vi "Consumer.vi"(8 "error in (no error)":errorcluster, 9 "Data":variant, 10 "Case ID":string, 11 "Tamer in":refnum<class "Tamer.lvclass">=refnum) -> (0 "error out":errorcluster, 3 "Tamer out":refnum<class "Tamer.lvclass">)   [LabVIEW 2020, in "CIRCUS_uServices.lvlib" / "Tamer.lvlib" / "Tamer.lvclass"]
uses:
  Tamer.lvclass
  Tamer Consumer Case Selector.ctl
  Run Utilities/TypeDefs/Messages/Schedule Message - Standard.ctl
  Run Utilities/Run Utilities.lvlib
  Run Utilities/TypeDefs/Return Code.ctl
  Run Utilities/TypeDefs/Messages/Banana Message.ctl
  Internatl Banana.ctl
  Tamer GV.vi
  TALOS/TALOS_PPL.lvlibp
  TALOS/TALOS_PPL.lvlibp/Father of all uServices/Father of all uServices/Father of all uServices.lvclass
  TALOS/TALOS_PPL.lvlibp/Guardian/Guardian/Requests.ctl
  TALOS/TALOS_PPL.lvlibp/Guardian/Guardian/Guardian.lvclass
  TALOS/TALOS_PPL.lvlibp/Ancestor/Ancestor/Infinite Message Selector.ctl
  TALOS/TALOS_PPL.lvlibp/Ancestor/Ancestor/Ancestor.lvclass
  TALOS/TALOS_PPL.lvlibp/Support VIs/Go-NoGo.ctl
  TALOS/TALOS_PPL.lvlibp/Support VIs/Global Constants.vi
  Run Utilities/TypeDefs/Messages/Monkey Status Message.ctl
  Run Utilities/TypeDefs/Monkey Status.ctl
  Run Utilities/TypeDefs/Script Checker Result.ctl
  Run Utilities/TypeDefs/Messages/Script Checker Message.ctl
  Run Utilities/TypeDefs/Synchronize FPGA Cluster.ctl
  Run Utilities/TypeDefs/Messages/Schedule Message - Parallel.ctl
  Stop Message.ctl
  Link Chain GUI.ctl
  Monkey Summary.ctl
  TALOS/TALOS_PPL.lvlibp/Father of all uServices/Father of all uServices/Children Methods/Get GUI Item Value - Variant.vi
  Run Utilities/Schedule/Schedule.lvclass
  C:/Users/marco/Documents/GitHub_Lab/CIRCUS/TALOS/TALOS_PPL.lvlibp/Father of all uServices/Father of all uServices/Father of all uServices.lvclass
  C:/Users/marco/Documents/GitHub_Lab/CIRCUS/TALOS/TALOS_PPL.lvlibp/Ancestor/Ancestor/Ancestor.lvclass
  C:/Users/marco/Documents/GitHub_Lab/CIRCUS/TALOS/Actor Framework.lvlibp/1abvi3w/vi.lib/ActorFramework/Actor/Actor.lvclass
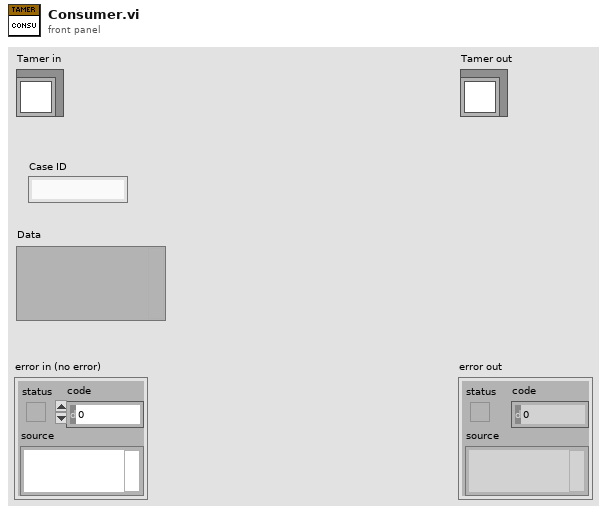
[diagram p1: front panel]
types:
  T1 = typedef "CIRCUS_uServices.lvlib/Tamer.lvlib/Tamer.lvclass/Tamer Consumer Case Selector.ctl" = enum16{"New schedule", "Initiate RUN", "Parse Schedules", "Script Checker", "Banana after Quality Check", "Update Crit Lvl", "Propagate Banana", "Reply from Guardian", "Reply from uService", "Timeout of RUN", "uService Replies Check", "Update from Monkey", "Monkey Died", "Reschedule", "Rerun", "Stop DAQ", "Stop Schedule", "Skip Run", "Kill Process", "Update GV"}
  T2 = typedef "CIRCUS_uServices.lvlib/Run Utilities.lvlib/Schedule Message - Standard.ctl" = cluster{"Schedules":refnum<class "Schedule.lvclass">[]}
  T3 = typedef "CIRCUS_uServices.lvlib/Run Utilities.lvlib/Schedule Message - Parallel.ctl" = cluster{"Schedules":refnum<class "Schedule.lvclass">[], "Synchronised":T4[]}
  T4 = typedef "CIRCUS_uServices.lvlib/Run Utilities.lvlib/Synchronize FPGA Cluster.ctl" = cluster{"Status":bool, "FPGA Name":string}
  T5 = typedef "TALOS_PPL.lvlibp/Guardian.lvlib/Guardian.lvclass/Requests.ctl" = enum16{"Ready to Launch", "Start RUN", "Stop RUN", "Update DAQ Params", "Update Error Listbox", "Update Run Status", "Update Kasli Log", "Run Stopped with Errors", "Switch uS View"}
  T6 = typedef "TALOS_PPL.lvlibp/Go-NoGo.ctl" = cluster{"ID":string, "Status":bool, "Data":string[], "GUID":string}
  T7 = typedef "CIRCUS_uServices.lvlib/Run Utilities.lvlib/Script Checker Message.ctl" = cluster{"Monkey ID":string, "Script Checker Result":T8}
  T8 = typedef "CIRCUS_uServices.lvlib/Run Utilities.lvlib/Script Checker Result.ctl" = enum16{"Passed", "Failed", "Empty"}
  T9 = typedef "CIRCUS_uServices.lvlib/Run Utilities.lvlib/Banana Message.ctl" = cluster{"FPGA Name":string, "Return Code":T10}
  T10 = typedef "CIRCUS_uServices.lvlib/Run Utilities.lvlib/Return Code.ctl" = enum16{"All Good", "Retry", "Skip", "Skip All", "ABORT"}
  T11 = typedef "CIRCUS_uServices.lvlib/Tamer.lvlib/Tamer.lvclass/Internatl Banana.ctl" = cluster{"Process ID":string, "Return Code":T10}
  T12 = typedef "CIRCUS_uServices.lvlib/Tamer.lvlib/Tamer.lvclass/Stop Message.ctl" = cluster{"Gracefully":bool, "Process":string}
  T13 = typedef "TALOS_PPL.lvlibp/Ancestor.lvlib/Ancestor.lvclass/Infinite Message Selector.ctl" = enum16{"Start", "Stop", "Check", "Flush (Stop all)", "Init"}
  T14 = typedef "CIRCUS_uServices.lvlib/Run Utilities.lvlib/Monkey Status Message.ctl" = cluster{"Monkey ID":string, "Monkey Status":T15, "Scripts left":u32, "ETA":string, "Current Action":string, "Report from previous RUNs":string, "Skipped RUNs":refnum<class "Schedule.lvclass">}
  T15 = typedef "CIRCUS_uServices.lvlib/Run Utilities.lvlib/Monkey Status.ctl" = enum16{"Init", "Paused", "Ongoing", "Stopped", "Finished (no errors)", "Finished (with errors)"}
  T16 = typedef "CIRCUS_uServices.lvlib/Tamer.lvlib/Tamer.lvclass/Monkey Summary.ctl" = cluster{"Color":u32, "Status":T15, "Continuous":bool, "Scripts left":u32, "Scripts skipped":u32, "ETA":string, "Current Action":string, "Report from previous RUNs":string, "Monkey ID":string, "With DAQ?":bool, "Linked?":T17, "Paused":bool}
  T17 = typedef "CIRCUS_uServices.lvlib/Tamer.lvlib/Tamer.lvclass/Link Chain GUI.ctl" = bool
  T18 = typedef "CIRCUS_uServices.lvlib/Tamer.lvlib/Tamer.lvclass/Tamer Status.ctl" = cluster{"Monkeys on the Stage":T16[], "All Monkeys Idle":bool}
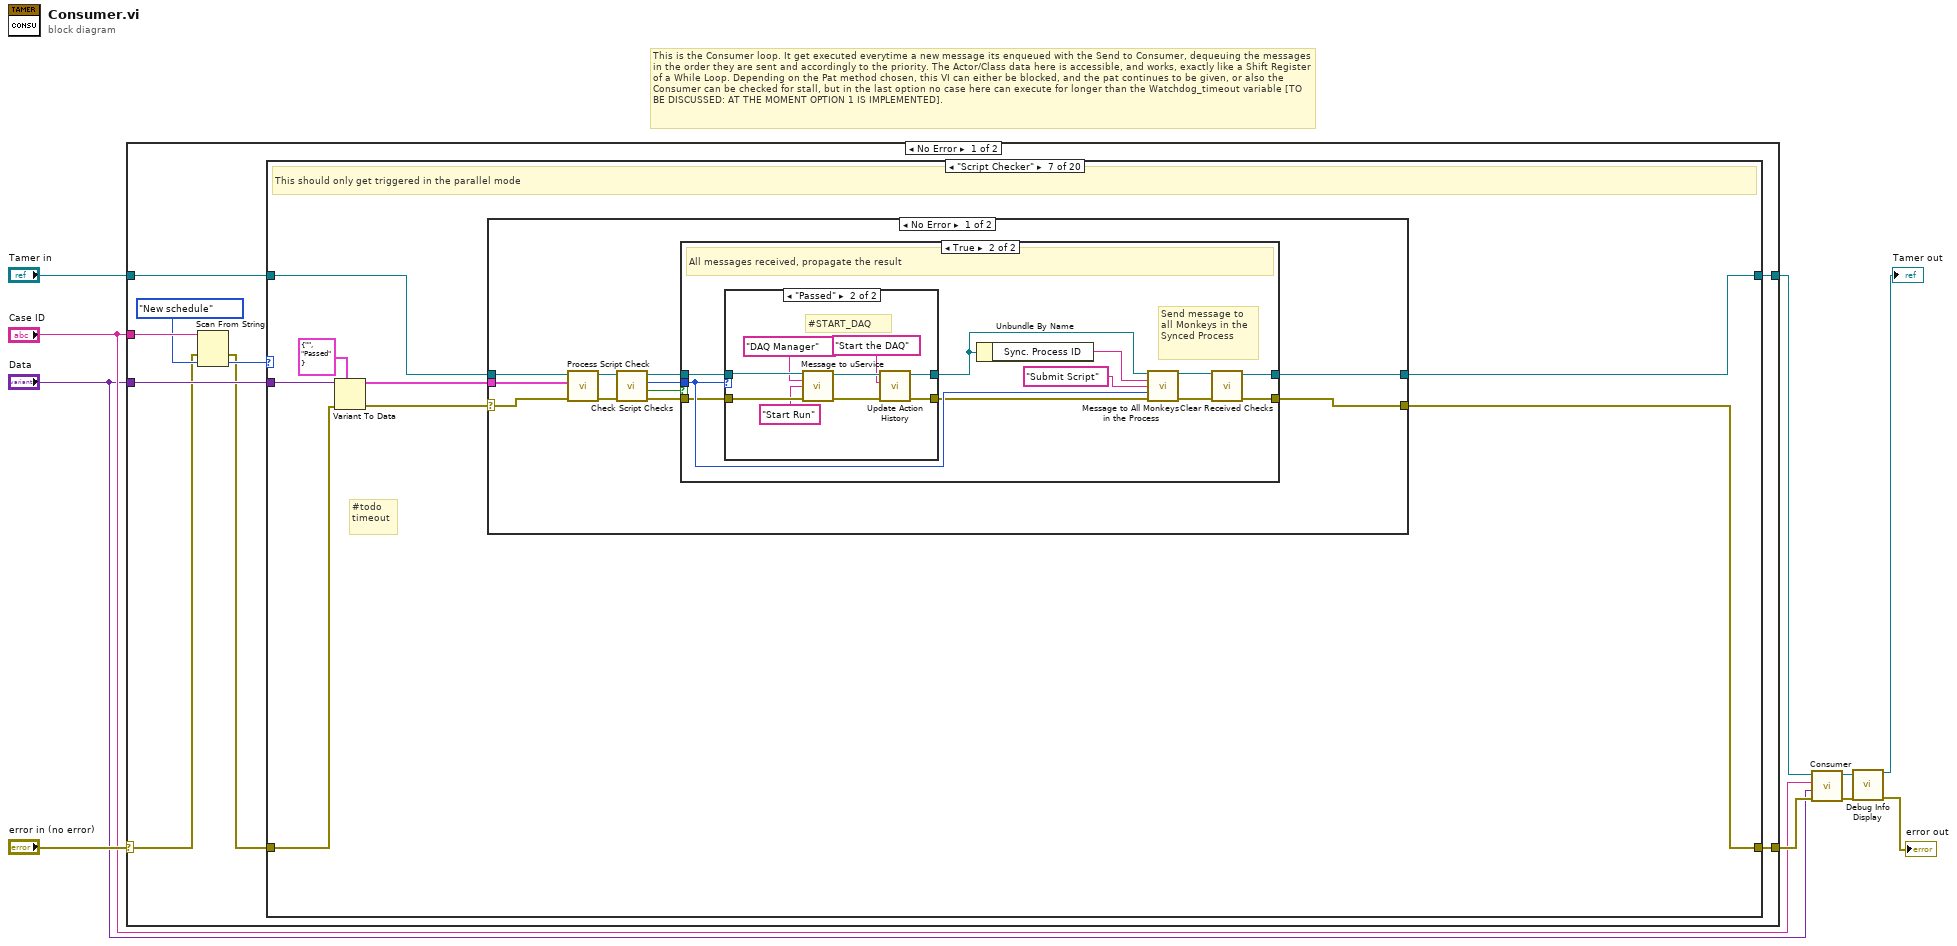
[diagram p0: block diagram]
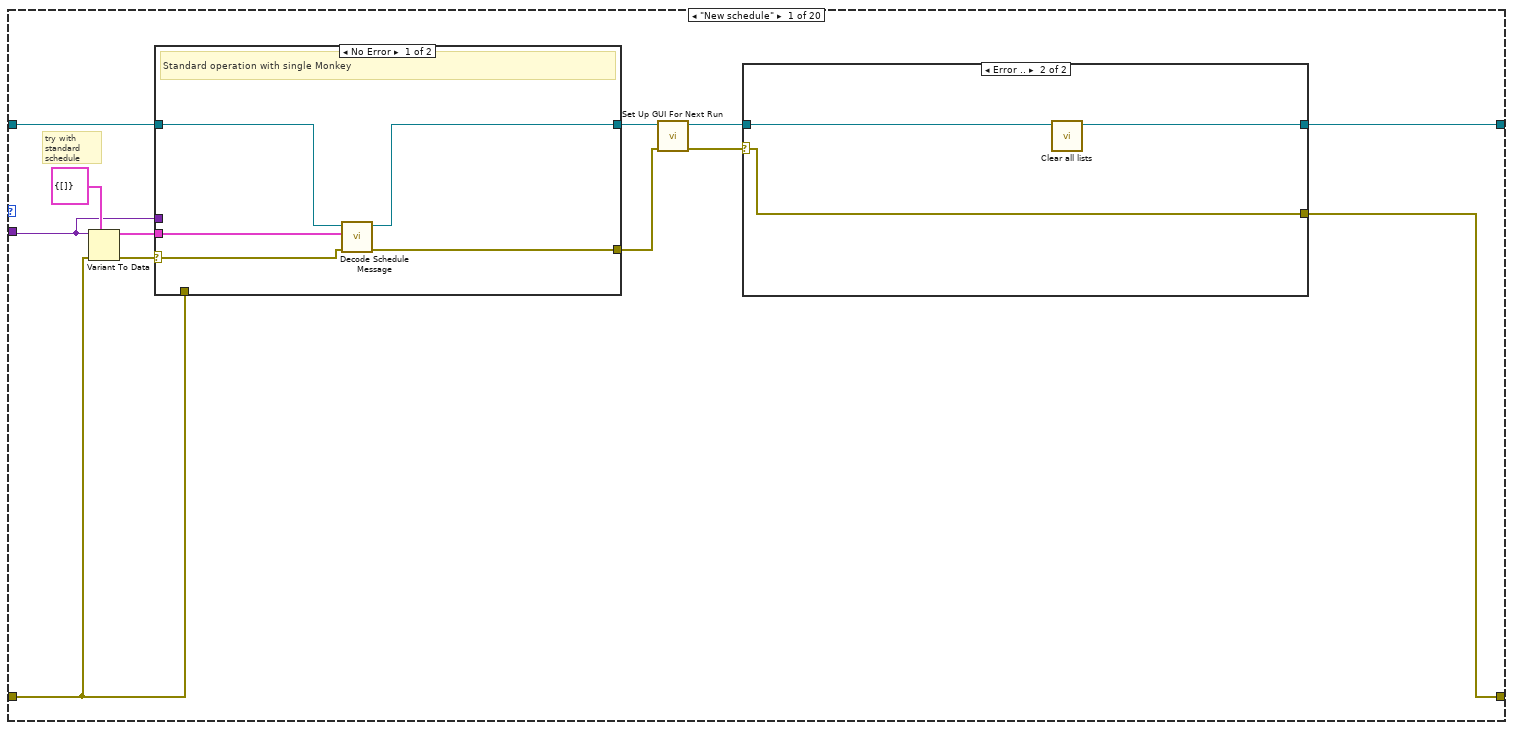
[diagram p2: hidden frame]
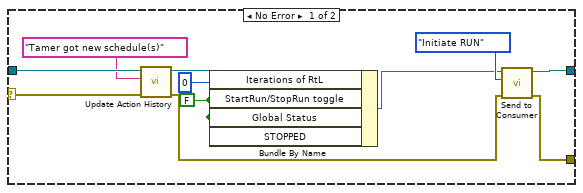
[diagram p3: hidden frame]
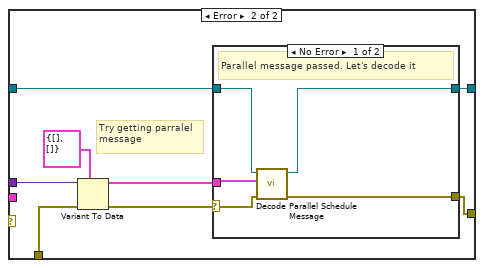
[diagram p4: hidden frame]
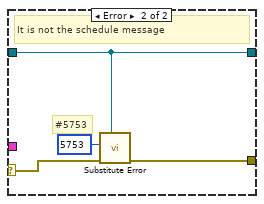
[diagram p5: hidden frame]
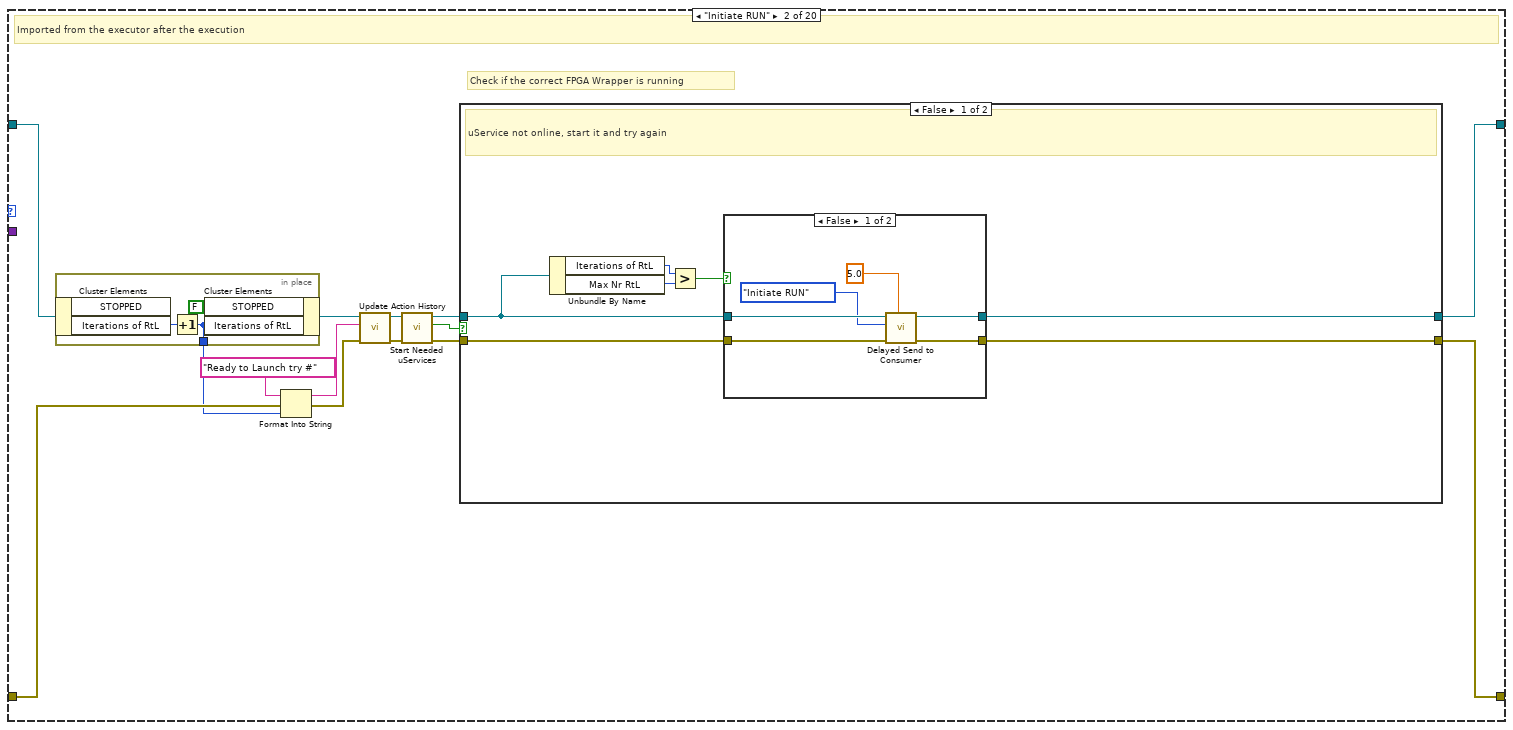
[diagram p6: hidden frame]
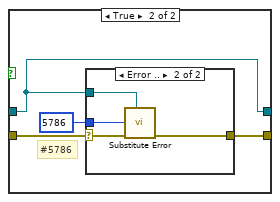
[diagram p7: hidden frame]
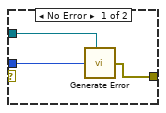
[diagram p8: hidden frame]
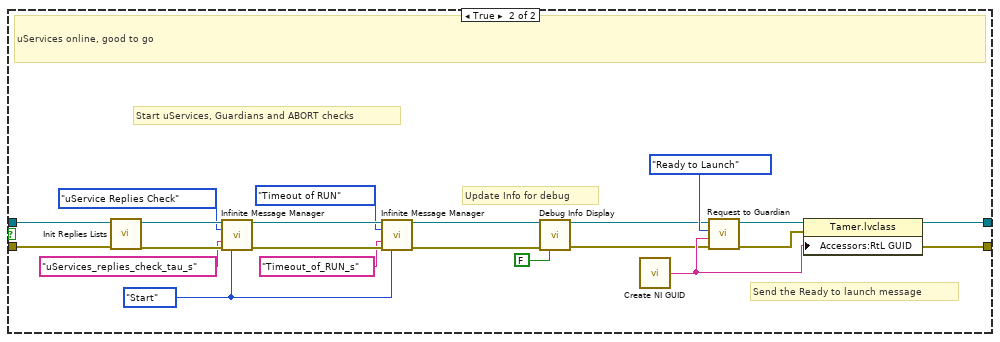
[diagram p9: hidden frame]
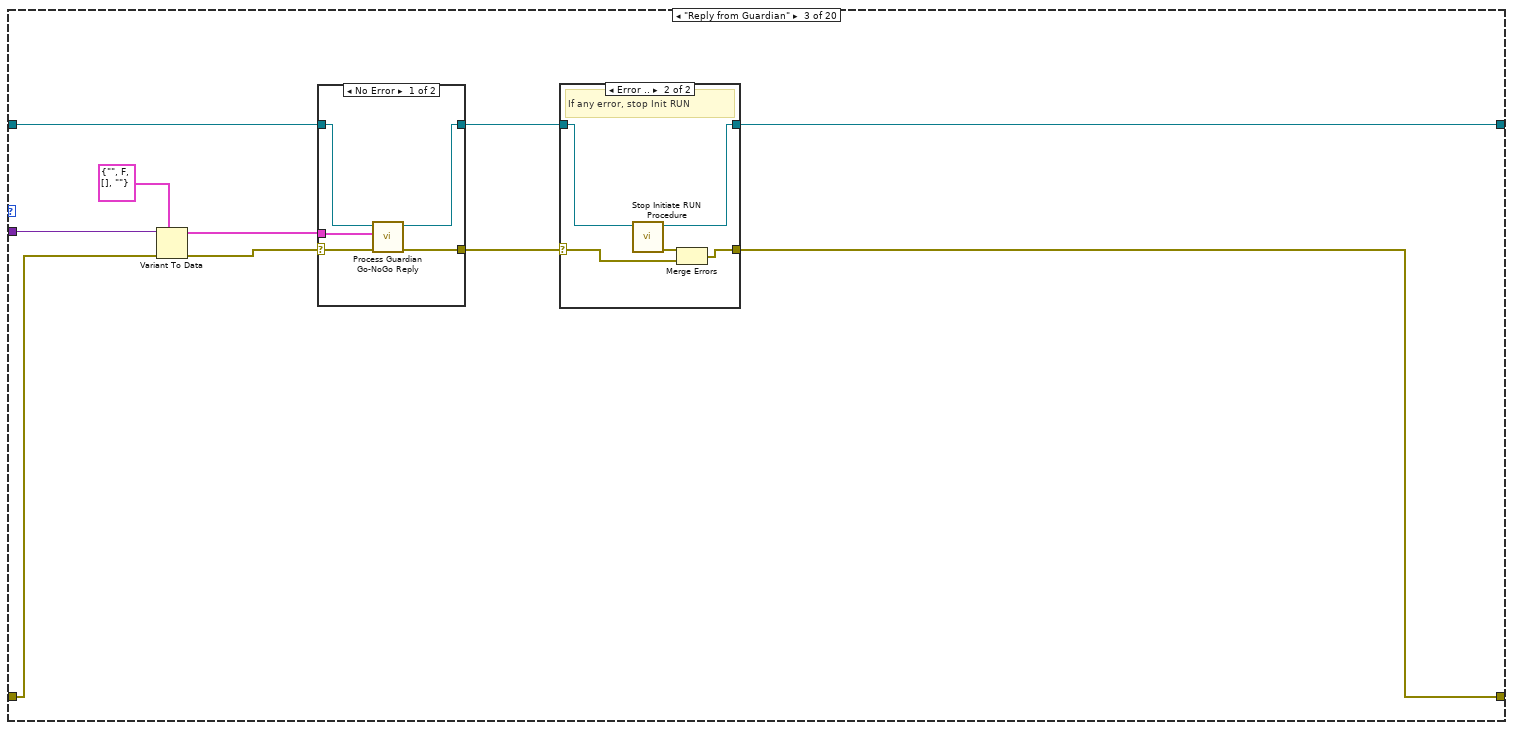
[diagram p10: hidden frame]
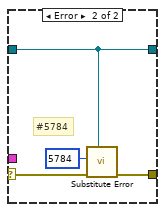
[diagram p12: hidden frame]
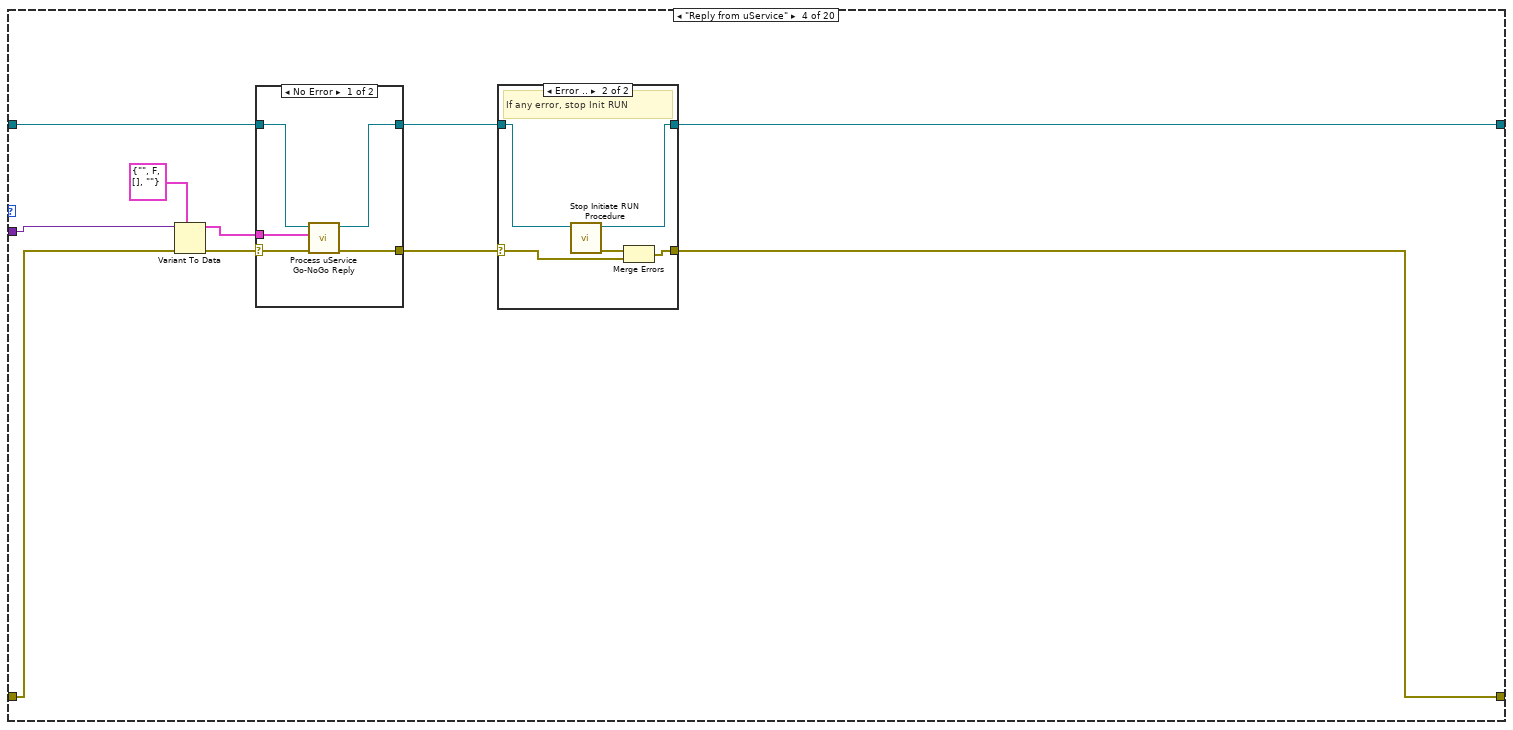
[diagram p13: hidden frame]
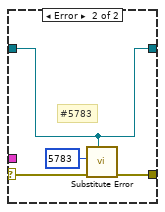
[diagram p15: hidden frame]
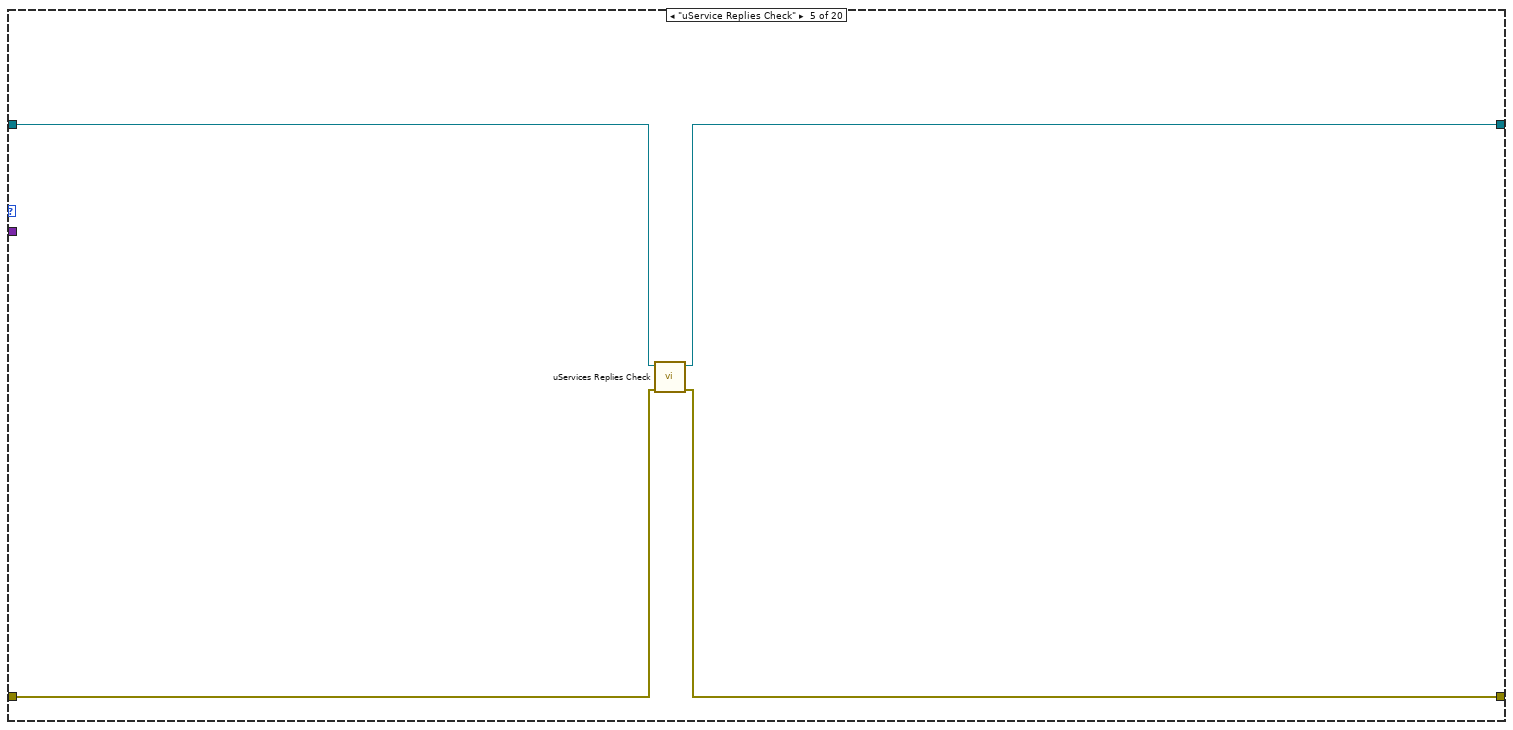
[diagram p16: hidden frame]
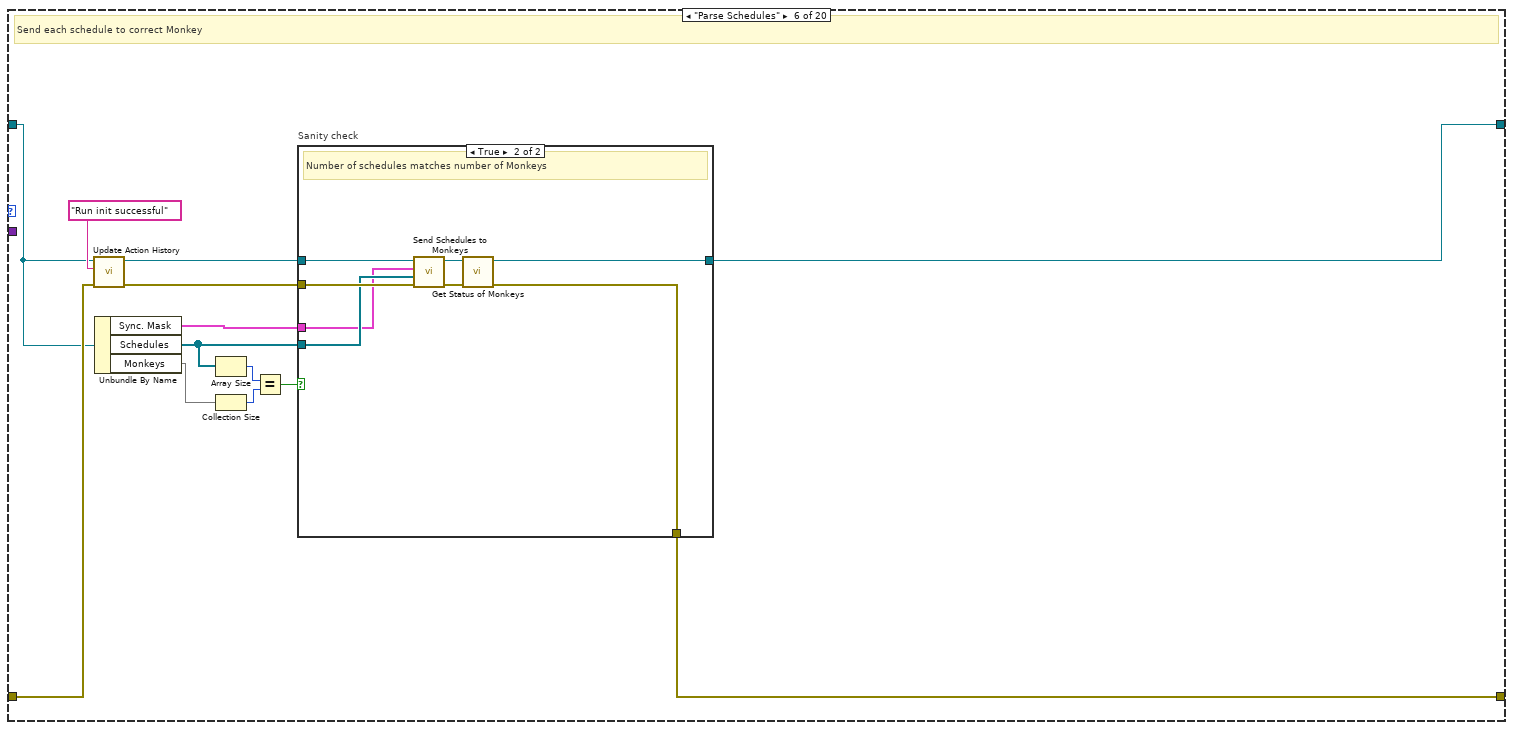
[diagram p17: hidden frame]
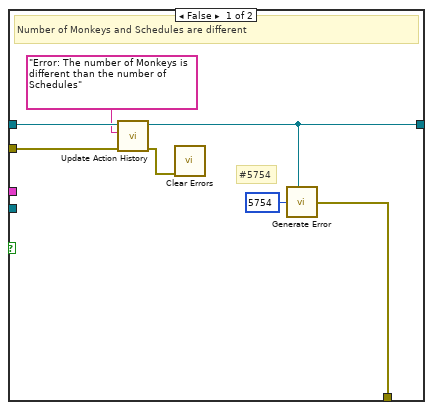
[diagram p18: hidden frame]
diagram:
  # "This is the Consumer loop. It get executed everytime a new message its enqueued with the Send to Consumer, dequeuing the messages in the order they are sent and accordingly to the priority. The Actor/Class data here is accessible, and works, exactly like a Shift Register of a While Loop. Depending on the Pat method chosen, this VI can either be blocked, and the pat continues to be given, or also the Consumer can be checked for stall, but in the last option no case here can execute for longer than the Watchdog_timeout variable [TO BE DISCUSSED: AT THE MOMENT OPTION 1 IS IMPLEMENTED]."
  n1 = case shown="No Error" "error in (no error)" {
    selector: "error in (no error)" -> [w12 w775]
    tunnel: [w18 w776] -> w7
    tunnel: "Tamer in" -> [w19 w776]
    tunnel: [w16 w775] -> w8
    tunnel: "Case ID" -> [w15 _]
    tunnel: "Data" -> [w17 _]
    frame No Error {
      n2 = Scan From String(input string=w15, error in=w12, default 1=Tamer_Consumer_Case_Selector."New schedule" ("Consumer Case Selector")) -> (error out=w11:errorcluster, output 1=w13:T1)  [unwired: 2 in, 2 out]
      n3 = case shown="\"Script Checker\"" w13 {
        tunnel: w19 -> [w26 w68 w136 w162 w183 w190 w217 w262 w329 w335 w354 w419 w435 w503 w543 w578 w627 w703 w767 w773]
        tunnel: [w21 w77 w135 w158 w184 w191 w215 w269 w328 w337 w364 w416 w437 w502 w562 w584 w631 w705 w764 w770] -> w18
        tunnel: w17 -> [w28 _ w134 w161 _ _ w222 w263 _ w341 w366 _ w440 w508 w549 w582 w632 w706 w763 _]
        tunnel: [w20 w76 w132 w159 w185 w197 w216 w268 w326 w336 w363 w417 w436 w501 w561 w586 w630 w704 w765 w769] -> w16
        tunnel: w11 -> [w27 w81 w133 w160 w186 w194 w220 w271 w327 w332 w365 w418 w438 w506 w550 w581 _ w707 w766 w772]
        frame "New schedule" {
          # "try with standard schedule"
          n4 = Variant To Data(error in=w27, type=T2 {"Schedules"=[]} ("Schedule message - parallel"), Variant=w28) -> (data=w29:T2, error out=w30:errorcluster)
          n5 = case shown="No Error" w30 {
            selector: w30 -> [w48 _]
            tunnel: w29 -> [w49 _]
            tunnel: w28 -> [_ w58]
            tunnel: w27 -> [_ w57]
            tunnel: w26 -> [w50 w53]
            tunnel: [w47 w52] -> w25
            tunnel: [w46 w51] -> w23
            frame No Error {
              # "Standard operation with single Monkey"
              n6 = call-dynamic "Decode Schedule Message.vi"("error in (no error)"=w48, "Schedule message"=w49, "Tamer in"=w50) -> ("error out"=w46:errorcluster, "Tamer out"=w47:refnum<class "Tamer.lvclass">)  [unwired: 7 in]
            }
            frame Error {
              # "Try getting parralel message"
              n7 = Variant To Data(error in=w57, type=T3 {"Schedules"=[], "Synchronised"=[]} ("Schedule message - parallel"), Variant=w58) -> (data=w54:T3, error out=w55:errorcluster)
              n8 = case shown="No Error" w55 {
                selector: w55 -> [w61 w66]
                tunnel: w54 -> [w63 _]
                tunnel: w53 -> [w62 w65]
                tunnel: [w60 w65] -> w52
                tunnel: [w59 w67] -> w51
                frame No Error {
                  # "Parallel message passed. Let's decode it"
                  n9 = call-dynamic "Decode Parallel Schedule Message.vi"("error in (no error)"=w61, "Schedule message - parallel"=w63, "Tamer in"=w62) -> ("error out"=w59:errorcluster, "Tamer out"=w60:refnum<class "Tamer.lvclass">)  [unwired: 7 in]
                }
                frame Error {
                  # "#5753"
                  # "It is not the schedule message"
                  n10 = call "Substitute Error.vi"("LabVIEW Object"=w65, "error in (no error)"=w66, "Error Code"=5753) -> ("error out"=w67:errorcluster)  [unwired: 8 in]
                }
              }
            }
          }
          n11 = call-dynamic "Set Up GUI For Next Run.vi"("error in (no error)"=w23, "Tamer in"=w25) -> ("error out"=w22:errorcluster, "Tamer out"=w24:refnum<class "Tamer.lvclass">)  [unwired: 8 in]
          n12 = case shown="Error .." w22 {
            selector: w22 -> [w37 w45]
            tunnel: [w34 w43] -> w21
            tunnel: w24 -> [w42 w44]
            tunnel: [w32 w45] -> w20
            frame No Error {
              w38 = FALSE ("StartRun/StopRun toggle")
              n13 = call-dynamic "Update Action History.vi"("error in (no error)"=w37, "Action"="Tamer got new schedule(s)", "Tamer in"=w42) -> ("error out"=w33:errorcluster, "Tamer out"=w40:refnum<class "Tamer.lvclass">)  [unwired: 7 in]
              n14 = Bundle By Name(cluster=w40, "Iterations of RtL"=u8 0, "StartRun/StopRun toggle"=w38, "Global Status"=w38, "STOPPED"=w38) -> (w35:refnum<class "Tamer.lvclass">)
              n15 = call "Send to Consumer.vi"("error in (no error)"=w33, "Case ID"=Tamer_Consumer_Case_Selector."Initiate RUN" ("Monkey Consumer Case Selector"), "uService Template in"=w35) -> ("error out"=w32:errorcluster, "uService Template out"=w34:refnum<class "Tamer.lvclass">)  [unwired: 7 in]
            }
            frame Error {
              n16 = call-dynamic "Clear all lists.vi"("Tamer in"=w44) -> ("Tamer out"=w43:refnum<class "Tamer.lvclass">)  [unwired: 9 in, 1 out]
            }
          }
        }
        frame "Initiate RUN" {
          # "Check if the correct FPGA Wrapper is running"
          # "Imported from the executor after the execution"
          n17 = in-place {
            in-place-border: [w82] -> w69
            n18 = in-place-cluster #1(w68) -> ("Iterations of RtL"=w84:u8)  [unwired: 1 out]
            n19 = Increment(x=w84) -> (x+1=w82:u8)
            n20 = in-place-cluster #1("STOPPED"=FALSE, "Iterations of RtL"=w82) -> (w73:refnum<class "Tamer.lvclass">)
          }
          n21 = Format Into String(initial string="Ready to Launch try #", error in=w81, w69) -> (resulting string=w71:string, error out=w70:errorcluster)  [unwired: 1 in]
          n22 = call-dynamic "Update Action History.vi"("error in (no error)"=w70, "Action"=w71, "Tamer in"=w73) -> ("error out"=w74:errorcluster, "Tamer out"=w75:refnum<class "Tamer.lvclass">)  [unwired: 7 in]
          n23 = call-dynamic "Start Needed uServices.vi"("error in (no error)"=w74, "Tamer in"=w75) -> ("error out"=w79:errorcluster, "All online?"=w80:bool, "Tamer out"=w78:refnum<class "Tamer.lvclass">)  [unwired: 7 in]
          n24 = case shown="False" w80 {
            tunnel: w79 -> [w89 w112]
            tunnel: w78 -> [w88 w113]
            tunnel: [w91 w115] -> w77
            tunnel: [w90 w114] -> w76
            frame False {
              # "uService not online, start it and try again"
              n25 = Unbundle By Name(w88) -> ("Iterations of RtL"=w87:u8, "Max Nr RtL"=w86:u8)
              n26 = Greater?(x=w87, y=w86) -> (0:w85:bool)
              n27 = case shown="False" w85 {
                tunnel: [w97 w99] -> w91
                tunnel: [w96 w100] -> w90
                tunnel: w88 -> [w95 w99]
                tunnel: w89 -> [w94 w101]
                frame False {
                  n28 = call "Delayed Send to Consumer.vi"("Seconds (5)"=5.0 ("Delay"), "error in (no error)"=w94, "Case ID"=Tamer_Consumer_Case_Selector."Initiate RUN" ("Tamer Consumer Case Selector"), "Father of all uServices in"=w95) -> ("error out"=w96:errorcluster, "Father of all uServices out"=w97:refnum<class "Tamer.lvclass">)  [unwired: 6 in]
                }
                frame True {
                  # "#5786"
                  n29 = case shown="Error .." w101 {
                    selector: w101 -> [_ w108]
                    tunnel: [w102 w107] -> w100
                    tunnel: w99 -> [w104 w106]
                    tunnel: 5786 -> [w103 w105]
                    frame No Error {
                      n30 = call "Generate Error.vi"("Class"=w104, "Error Code"=w103) -> ("error out"=w102:errorcluster)  [unwired: 5 in]
                    }
                    frame Error {
                      n31 = call "Substitute Error.vi"("LabVIEW Object"=w106, "error in (no error)"=w108, "Error Code"=w105) -> ("error out"=w107:errorcluster)  [unwired: 8 in]
                    }
                  }
                }
              }
            }
            frame True {
              w123 = Infinite_Message_Selector."Start" ("Infinite Message Selector")
              # "Start uServices, Guardians and ABORT checks"
              # "Update Info for debug"
              # "Send the Ready to launch message"
              # "uServices online, good to go"
              n32 = call "Init Replies Lists.vi"("error in (no error)"=w112, "Monkey in"=w113) -> ("error out"=w127:errorcluster, "Monkey out"=w128:refnum<class "Tamer.lvclass">)  [unwired: 8 in]
              n33 = call-dynamic "Infinite Message Manager.vi"("Father of all uServices in"=w128, "Consumer Case Selector"=Tamer_Consumer_Case_Selector."uService Replies Check" ("Monkey Consumer Case Selector"), "Tau parameter"="uServices_replies_check_tau_s" ("SV Name"), "error in (no error)"=w127, "Infinite Message Selector"=w123) -> ("Father of all uServices out"=w125:refnum<class "Tamer.lvclass">, "error out"=w124:errorcluster)  [unwired: 8 in, 1 out]
              n34 = call-dynamic "Infinite Message Manager.vi"("Father of all uServices in"=w125, "Consumer Case Selector"=Tamer_Consumer_Case_Selector."Timeout of RUN" ("Monkey Consumer Case Selector"), "Tau parameter"="Timeout_of_RUN_s" ("SV Name"), "error in (no error)"=w124, "Infinite Message Selector"=w123) -> ("Father of all uServices out"=w119:refnum<class "Tamer.lvclass">, "error out"=w116:errorcluster)  [unwired: 8 in, 1 out]
              n35 = call-dynamic "Debug Info Display.vi"("Tamer in"=w119, "error in (no error)"=w116, "Do not clear"=FALSE) -> ("Tamer out"=w118:refnum<class "Tamer.lvclass">, "error out"=w117:errorcluster)  [unwired: 11 in]
              n36 = call <vilib>:"Create NI GUID.vi"() -> ("NI GUID"=w120:string)
              n37 = call "Request to Guardian.vi"("error in (no error)"=w117, "Data"=w120, "Requests"=Requests."Ready to Launch", "Father of all uServices in"=w118) -> ("error out"=w110:errorcluster, "Father of all uServices out"=w130:refnum<class "Tamer.lvclass">)  [unwired: 6 in]
              n38 = property class="Tamer.lvclass"(reference=w130, error in=w110, "Accessors:RtL GUID"=w120) -> (reference out=w115:refnum<class "Tamer.lvclass">, error out=w114:errorcluster)
            }
          }
        }
        frame "Reply from Guardian" {
          n39 = Variant To Data(error in=w133, type=T6 {"ID"="", "Status"=FALSE, "Data"=[], "GUID"=""} ("Go-NoGo"), Variant=w134) -> (data=w138:T6, error out=w139:errorcluster)
          n40 = case shown="No Error" w139 {
            selector: w139 -> [w152 w155]
            tunnel: [w151 w156] -> w140
            tunnel: w138 -> [w150 _]
            tunnel: w136 -> [w149 w153]
            tunnel: [w148 w153] -> w137
            frame No Error {
              n41 = call "Process Guardian Go-NoGo Reply.vi"("error in (no error)"=w152, "Go-NoGo"=w150, "Tamer in"=w149) -> ("error out"=w151:errorcluster, "Tamer out"=w148:refnum<class "Tamer.lvclass">)  [unwired: 7 in]
            }
            frame Error {
              # "#5784"
              n42 = call "Substitute Error.vi"("LabVIEW Object"=w153, "error in (no error)"=w155, "Error Code"=5784) -> ("error out"=w156:errorcluster)  [unwired: 8 in]
            }
          }
          n43 = case shown="Error .." w140 {
            selector: w140 -> [w142 w144]
            tunnel: [w142 w143] -> w132
            tunnel: [w141 w147] -> w135
            tunnel: w137 -> [w141 w146]
            frame No Error {
              # "All good!"
            }
            frame Error {
              # "If any error, stop Init RUN"
              n44 = call "Stop Initiate RUN Procedure.vi"("Tamer in"=w146) -> ("error out"=w145:errorcluster, "Tamer out"=w147:refnum<class "Tamer.lvclass">)  [unwired: 9 in]
              n45 = Merge Errors(w145, w144) -> (w143:errorcluster)
            }
          }
        }
        frame "Reply from uService" {
          n46 = Variant To Data(error in=w160, type=T6 {"ID"="", "Status"=FALSE, "Data"=[], "GUID"=""} ("Go-NoGo"), Variant=w161) -> (data=w166:T6, error out=w165:errorcluster)
          n47 = case shown="No Error" w165 {
            selector: w165 -> [w177 w181]
            tunnel: w166 -> [w178 _]
            tunnel: [w176 w182] -> w163
            tunnel: [w175 w179] -> w164
            tunnel: w162 -> [w174 w179]
            frame No Error {
              n48 = call "Process uService Go-NoGo Reply.vi"("error in (no error)"=w177, "Go-NoGo"=w178, "Tamer in"=w174) -> ("error out"=w176:errorcluster, "Tamer out"=w175:refnum<class "Tamer.lvclass">)  [unwired: 7 in]
            }
            frame Error {
              # "#5783"
              n49 = call "Substitute Error.vi"("LabVIEW Object"=w179, "error in (no error)"=w181, "Error Code"=5783) -> ("error out"=w182:errorcluster)  [unwired: 8 in]
            }
          }
          n50 = case shown="Error .." w163 {
            selector: w163 -> [w168 w169]
            tunnel: w164 -> [w167 w173]
            tunnel: [w168 w170] -> w159
            tunnel: [w167 w172] -> w158
            frame No Error {
              # "All good!"
            }
            frame Error {
              # "If any error, stop Init RUN"
              n51 = call "Stop Initiate RUN Procedure.vi"("Tamer in"=w173) -> ("error out"=w171:errorcluster, "Tamer out"=w172:refnum<class "Tamer.lvclass">)  [unwired: 9 in]
              n52 = Merge Errors(w171, w169) -> (w170:errorcluster)
            }
          }
        }
        frame "uService Replies Check" {
          n53 = call "uServices Replies Check.vi"("error in (no error)"=w186, "Tamer in"=w183) -> ("error out"=w185:errorcluster, "Tamer out"=w184:refnum<class "Tamer.lvclass">)  [unwired: 8 in]
        }
        frame "Parse Schedules" {
          # "Send each schedule to correct Monkey"
          n54 = call-dynamic "Update Action History.vi"("error in (no error)"=w194, "Action"="Run init successful", "Tamer in"=w190) -> ("error out"=w192:errorcluster, "Tamer out"=w195:refnum<class "Tamer.lvclass">)  [unwired: 7 in]
          n55 = Unbundle By Name(w190) -> ("Sync. Mask"=w199:T4[], "Schedules"=w198:refnum<class "Schedule.lvclass">[], "Monkeys"=w188:map{string, string[]})
          n56 = Array Size(array=w198) -> (size(s)=w189:i32)
          n57 = Collection Size(1:w188) -> (0:w187:i32)
          n58 = Equal?(x=w189, y=w187) -> (x = y?=w196:bool)
          n59 = case "Sanity check" shown="True" w196 {
            tunnel: w199 -> [_ w211]
            tunnel: w195 -> [w204 w213]
            tunnel: w198 -> [_ w212]
            tunnel: [w205 w207] -> w197
            tunnel: w192 -> [w203 w214]
            tunnel: [w200 w209] -> w191
            frame False {
              # "#5754"
              # "Number of Monkeys and Schedules are different"
              n60 = call-dynamic "Update Action History.vi"("error in (no error)"=w203, "Action"="Error: The number of Monkeys is different than the number of Schedules", "Tamer in"=w204) -> ("error out"=w201:errorcluster, "Tamer out"=w200:refnum<class "Tamer.lvclass">)  [unwired: 7 in]
              n61 = call <vilib>:"Clear Errors.vi"("error in (no error)"=w201) -> ()  [unwired: 5 in, 2 out]
              n62 = call "Generate Error.vi"("Class"=w200, "Error Code"=5754) -> ("error out"=w205:errorcluster)  [unwired: 5 in]
            }
            frame True {
              # "Number of schedules matches number of Monkeys"
              n63 = call "Send Schedules to Monkeys.vi"("error in (no error)"=w214, "Schedules"=w212, "Sync. Mask"=w211, "Tamer in"=w213) -> ("error out"=w208:errorcluster, "Tamer out"=w210:refnum<class "Tamer.lvclass">)  [unwired: 6 in]
              n64 = call-dynamic "Get Status of Monkeys.vi"("error in (no error)"=w208, "Tamer in"=w210) -> ("error out"=w207:errorcluster, "Tamer out"=w209:refnum<class "Tamer.lvclass">)  [unwired: 7 in, 1 out]
            }
          }
        }
        frame "Script Checker" {
          # "#todo\ntimeout"
          # "This should only get triggered in the parallel mode"
          n65 = Variant To Data(error in=w220, type=T7 {"Monkey ID"="", "Script Checker Result"=enum."Passed"} ("Message"), Variant=w222) -> (data=w218:T7, error out=w219:errorcluster)
          n66 = case shown="No Error" w219 {
            selector: w219 -> [w233 w261]
            tunnel: w218 -> [w224 _]
            tunnel: w217 -> [w225 w259]
            tunnel: [w223 w260] -> w216
            tunnel: [w226 w259] -> w215
            frame No Error {
              n67 = call-dynamic "Process Script Check.vi"("error in (no error)"=w233, "Message"=w224, "Tamer in"=w225) -> ("error out"=w231:errorcluster, "Tamer out"=w232:refnum<class "Tamer.lvclass">)  [unwired: 7 in]
              n68 = call-dynamic "Check Script Checks.vi"("error in (no error)"=w231, "Tamer in"=w232) -> ("error out"=w229:errorcluster, "Send Result?"=w230:bool, "Script Checker Result"=w228:T8, "Tamer out"=w227:refnum<class "Tamer.lvclass">)  [unwired: 6 in]
              n69 = case shown="True" w230 {
                tunnel: w229 -> [w234 w239]
                tunnel: w228 -> [_ w244]
                tunnel: w227 -> [w235 w238]
                tunnel: [w234 w241] -> w223
                tunnel: [w235 w240] -> w226
                frame False {
                  # "Waiting for some responses"
                }
                frame True {
                  # "Send message to all Monkeys in the Synced Process"
                  # "All messages received, propagate the result"
                  n70 = case shown="\"Passed\"" w244 {
                    tunnel: w238 -> [w248 w251]
                    tunnel: w239 -> [w247 w254]
                    tunnel: [w247 w253] -> w236
                    tunnel: [w248 w252] -> w237
                    frame Default {
                    }
                    frame "Passed" {
                      # "#START_DAQ"
                      n71 = call "Message to uService.vi"("Father of all uServices in"=w251, "uService ID"="DAQ Manager", "Message"="Start Run", "error in (no error)"=w254) -> ("Father of all uServices out"=w256:refnum<class "Tamer.lvclass">, "error out"=w257:errorcluster)  [unwired: 10 in]
                      n72 = call-dynamic "Update Action History.vi"("error in (no error)"=w257, "Action"="Start the DAQ", "Tamer in"=w256) -> ("error out"=w253:errorcluster, "Tamer out"=w252:refnum<class "Tamer.lvclass">)  [unwired: 7 in]
                    }
                  }
                  n73 = Unbundle By Name(w237) -> ("Sync. Process ID"=w245:string)
                  n74 = call-dynamic "Message to All Monkeys in the Process.vi"("Tamer in"=w237, "Process ID"=w245, "Message"="Submit Script", "Data"=w244, "error in (no error)"=w236) -> ("Tamer out"=w243:refnum<class "Tamer.lvclass">, "error out"=w242:errorcluster)  [unwired: 9 in]
                  n75 = call-dynamic "Clear Received Checks.vi"("error in (no error)"=w242, "Tamer in"=w243) -> ("error out"=w241:errorcluster, "Tamer out"=w240:refnum<class "Tamer.lvclass">)  [unwired: 8 in]
                }
              }
            }
            frame Error {
              # "#5207"
              n76 = call "Substitute Error.vi"("LabVIEW Object"=w259, "error in (no error)"=w261, "Error Code"=5207) -> ("error out"=w260:errorcluster)  [unwired: 8 in]
            }
          }
        }
        frame "Banana after Quality Check" {
          # "This case is needed to avoid the race condition of an error getting enqueued immediately after the Run is finished: the Monkey would then skip the Criticality Level associated to that error (and, by the way, using it in the subsequent Run). In this way, the \"What to do next\" will be enqued after any - reasonably - possible \"Error Criticality\" message from the Error Manager."
          n77 = Variant To Data(error in=w271, type=T9 {"FPGA Name"="", "Return Code"=enum."All Good"} ("Cluster"), Variant=w263) -> (data=w266:T9, error out=w267:errorcluster)
          n78 = case shown="No Error" w267 {
            selector: w267 -> [w272 _]
            tunnel: w266 -> [w273 _]
            tunnel: [w273 w282] -> w265
            tunnel: [w272 w278] -> w264
            tunnel: w263 -> [_ w281]
            tunnel: w262 -> [_ w277]
            frame No Error {
            }
            frame Error {
              n79 = Variant To Data(type="", Variant=w281) -> (data=w276:string, error out=w279:errorcluster)  [unwired: 1 in]
              n80 = call-dynamic "Get FPGA Name From Monkey ID.vi"("error in (no error)"=w279, "Monkey ID"=w276, "Tamer in"=w277) -> ("error out"=w278:errorcluster, "FPGA Name"=w275:string)  [unwired: 6 in, 1 out]
              n81 = Bundle By Name(cluster=T9 {"FPGA Name"="", "Return Code"=enum."All Good"} ("Cluster"), "Return Code"=Return_Code."Skip", "FPGA Name"=w275) -> (w282:T9)
            }
          }
          n82 = case shown="No Error" w264 {
            selector: w264 -> [w291 w320]
            tunnel: [w287 w324] -> w269
            tunnel: [w284 w323] -> w268
            tunnel: w262 -> [w286 w324]
            tunnel: w265 -> [w285 _]
            frame No Error {
              n83 = call-dynamic "Process Banana Message.vi"("error in (no error)"=w291, "Message"=w285, "Tamer in"=w286) -> ("error out"=w292:errorcluster, "Propagate Banana?"=w290:bool, "Internal Banana"=w288:T11, "Tamer out"=w289:refnum<class "Tamer.lvclass">)  [unwired: 5 in]
              n84 = case shown="True" w290 {
                tunnel: w289 -> [w294 w304]
                tunnel: w292 -> [w293 w305]
                tunnel: w288 -> [_ w295]
                tunnel: [w294 w299] -> w287
                tunnel: [w293 w297] -> w284
                frame False {
                  # "Do not propagate Banana (maybe not all Monkeys finished, or there was ABORT)"
                }
                frame True {
                  # "avoid enqueuing a new script before the previous one has finished"
                  # "Let's Propagate with a delay"
                  n85 = Unbundle By Name(w304) -> ("Sync. Process ID"=w303:string)
                  n86 = Unbundle By Name(w295) -> ("Process ID"=w302:string)
                  n87 = Equal?(x=w303, y=w302) -> (x = y?=w301:bool)
                  n88 = case shown="True" w301 {
                    tunnel: w305 -> [w309 w318]
                    tunnel: [w312 w319] -> w300
                    tunnel: [w307 w318] -> w298
                    tunnel: w304 -> [w311 w319]
                    tunnel: [w313 1.0] -> w306
                    frame True {
                      # "#STOP_DAQ"
                      # "In synchronised we need to stop DAQ"
                      n89 = call "Send to Consumer.vi"("error in (no error)"=w309, "Case ID"=Tamer_Consumer_Case_Selector."Stop DAQ" ("Consumer Case Selector"), "uService Template in"=w311) -> ("error out"=w308:errorcluster, "uService Template out"=w312:refnum<class "Tamer.lvclass">)  [unwired: 7 in]
                      n90 = call "TALOS Config Param.vi"("error in (no error)"=w308, "Parameter Name"="Stop_DAQ_Delay_s") -> ("error out"=w307:errorcluster, "Output"=w315:string)  [unwired: 8 in]
                      n91 = Fract/Exp String To Number(string=w315, default (0 dbl)=10.0 ("default (0 DBL)")) -> (number=w313:dbl)  [unwired: 2 in, 1 out]
                    }
                    frame False {
                      # "Not synchronised, just send it"
                    }
                  }
                  n92 = call "Delayed Send to Consumer.vi"("Seconds (5)"=w306, "error in (no error)"=w298, "Data"=w295, "Case ID"=Tamer_Consumer_Case_Selector."Propagate Banana" ("Consumer Case Selector"), "Father of all uServices in"=w300) -> ("error out"=w297:errorcluster, "Father of all uServices out"=w299:refnum<class "Tamer.lvclass">)  [unwired: 5 in]
                }
              }
            }
            frame Error {
              # "#5207"
              n93 = call "Substitute Error.vi"("LabVIEW Object"=w324, "error in (no error)"=w320, "Error Code"=5207, "Optional String"="Wrong banana message!") -> ("error out"=w323:errorcluster)  [unwired: 7 in]
            }
          }
        }
        frame "Stop DAQ" {
          # "#STOP_DAQ"
          n94 = call "Message to uService.vi"("Father of all uServices in"=w329, "uService ID"="DAQ Manager", "Message"="Stop Run", "error in (no error)"=w327) -> ("Father of all uServices out"=w328:refnum<class "Tamer.lvclass">, "error out"=w326:errorcluster)  [unwired: 10 in]
        }
        frame "Propagate Banana" {
          # "By default, I mean"
          # "#Stop or ABORT?"
          # "Send Processed Banana to each Monkey that needs to receive it"
          n95 = call-dynamic "Update Action History.vi"("error in (no error)"=w332, "Action"="Propagate Banana", "Tamer in"=w335) -> ("error out"=w333:errorcluster, "Tamer out"=w334:refnum<class "Tamer.lvclass">)  [unwired: 7 in]
          n96 = Variant To Data(error in=w333, type=T11 {"Process ID"="", "Return Code"=enum."All Good"} ("Internal Banana"), Variant=w341) -> (data=w339:T11, error out=w338:errorcluster)
          n97 = case shown="No Error" w338 {
            selector: w338 -> [w346 w353]
            tunnel: w339 -> [w349 _]
            tunnel: [w345 w351] -> w337
            tunnel: [w344 w352] -> w336
            tunnel: w334 -> [w342 w351]
            frame No Error {
              n98 = Unbundle By Name(w349) -> ("Process ID"=w348:string, "Return Code"=w347:T10)
              n99 = call-dynamic "Message to All Monkeys in the Process.vi"("Tamer in"=w342, "Process ID"=w348, "Message"="B4N4N4", "Data"=w347, "error in (no error)"=w346) -> ("Tamer out"=w345:refnum<class "Tamer.lvclass">, "error out"=w344:errorcluster)  [unwired: 9 in]
            }
            frame Error {
              # "#5207"
              n100 = call "Substitute Error.vi"("LabVIEW Object"=w351, "error in (no error)"=w353, "Error Code"=5207) -> ("error out"=w352:errorcluster)  [unwired: 8 in]
            }
          }
        }
        frame "Update Crit Lvl" {
          # "Volpe: it is correct to forward the criticality level to each Monkey and let them handle it, because if they are running async, they need to independently choose what to do"
          # "If there was an error in variant to data, it means that the variant was empty: no specific error was provided. Ignore that error"
          # "Send Criticality level to every Running Monkey. so it knows"
          n101 = Variant To Data(error in=w365, type=u8 0, Variant=w366) -> (data=w361:u8, error out=w362:errorcluster)
          n102 = global read "Global Constants.vi" "ABORT Crt Lvl"() -> (w357:u8)
          n103 = case shown="No Error" w362 {
            selector: w362 -> [w409 w414]
            tunnel: w361 -> [w410 _]
            tunnel: [w410 w411] -> w360
            tunnel: [w409 w413] -> w359
            tunnel: w357 -> [_ w412]
            frame No Error {
            }
            frame Error {
              n104 = call <vilib>:"Clear Errors.vi"("error in (no error)"=w414) -> ("error out"=w413:errorcluster)  [unwired: 5 in, 1 out]
              n105 = Decrement(x=w412) -> (x-1=w411:u8)
            }
          }
          n106 = case shown="No Error" w359 {
            selector: w359 -> [w394 w408]
            tunnel: w360 -> [w397 _]
            tunnel: [w393 w407] -> w356
            tunnel: [w392 w405] -> w355
            tunnel: w357 -> [w391 w405]
            tunnel: w354 -> [w390 w404]
            frame No Error {
              n107 = In Range and Coerce(upper limit=w391, x=w397, lower limit=u8 0) -> (In Range?=w395:bool)  [unwired: 1 out]
              n108 = case shown="False" w395 {
                tunnel: w397 -> [_ w403]
                tunnel: w394 -> [_ w402]
                tunnel: [w401 w402] -> w393
                tunnel: [w399 w403] -> w392
                tunnel: w391 -> [w399 _]
                tunnel: w390 -> [w398 _]
                frame False {
                  # "#5788"
                  n109 = call "Generate Error.vi"("Class"=w398, "Error Code"=5788) -> ("error out"=w401:errorcluster)  [unwired: 5 in]
                }
                frame True {
                  # "All good!"
                }
              }
            }
            frame Error {
              # "#5788"
              n110 = call "Substitute Error.vi"("LabVIEW Object"=w404, "error in (no error)"=w408, "Error Code"=5788) -> ("error out"=w407:errorcluster)  [unwired: 8 in]
            }
          }
          n111 = case shown="3" w355 {
            selector: w355 -> [w367 _ _]
            tunnel: w354 -> [w371 w382 w385]
            tunnel: w356 -> [w370 w380 w388]
            tunnel: [w368 w374 w384] -> w364
            tunnel: [w369 w379 w387] -> w363
            frame Default {
              n112 = call-dynamic "Send Error Criticality.vi"("error in (no error)"=w370, "Crit. Level"=w367, "Tamer in"=w371) -> ("error out"=w369:errorcluster, "Tamer out"=w368:refnum<class "Tamer.lvclass">)  [unwired: 5 in]
            }
            frame 3 {
              # "To stop gracefully all the running processes"
              n113 = call "Send to Consumer.vi"("Data"=T12 {"Gracefully"=TRUE, "Process"="ALL"} ("cluster"), "Case ID"=Tamer_Consumer_Case_Selector."Stop Schedule" ("Monkey Consumer Case Selector"), "uService Template in"=w382) -> ("error out"=w375:errorcluster, "uService Template out"=w376:refnum<class "Tamer.lvclass">)  [unwired: 7 in]
              n114 = call "Request to Guardian.vi"("error in (no error)"=w375, "Data"=FALSE, "Requests"=Requests."Run Stopped with Errors", "Father of all uServices in"=w376) -> ("error out"=w373:errorcluster, "Father of all uServices out"=w374:refnum<class "Tamer.lvclass">)  [unwired: 6 in]
              n115 = Merge Errors(w373, w380) -> (w379:errorcluster)
            }
            frame 4 {
              # "Let safe mode do the work"
              n116 = call "Raise ABORT.vi"("error in"=w388, "ABORT?"=TRUE) -> ("error out"=w387:errorcluster)  [unwired: 9 in]
              n117 = call "Request to Guardian.vi"("Data"=FALSE, "Requests"=Requests."Run Stopped with Errors", "Father of all uServices in"=w385) -> ("Father of all uServices out"=w384:refnum<class "Tamer.lvclass">)  [unwired: 7 in, 1 out]
            }
          }
        }
        frame "Timeout of RUN" {
          # "Checks if someone has already stopped Timeout of RUN (but this message has already get enqueued): in case, do nothing, because it means that the RUN Init Procedure has completed successfully (albeit just in time). In case Timeout of RUN was still on, terminate the RUN Init Procedure and thow the timeout error."
          # "Stop the RUN Init Procedure and raise ABORT."
          n118 = call-dynamic "Infinite Message Manager.vi"("Father of all uServices in"=w419, "Consumer Case Selector"=Tamer_Consumer_Case_Selector."Timeout of RUN" ("Monkey Consumer Case Selector"), "Infinite Message Selector"=Infinite_Message_Selector."Check") -> ("Father of all uServices out"=w423:refnum<class "Tamer.lvclass">, "Exists?"=w422:bool, "error out"=w421:errorcluster)  [unwired: 10 in]
          n119 = case shown="True" w422 {
            tunnel: [w426 w432] -> w416
            tunnel: w423 -> [w426 w427]
            tunnel: [w425 w431] -> w424
            tunnel: w421 -> [w425 w429]
            frame False {
            }
            frame True {
              # "#5778"
              n120 = call "Substitute Error.vi"("LabVIEW Object"=w427, "error in (no error)"=w429, "Error Code"=5778) -> ("error out"=w428:errorcluster)  [unwired: 8 in]
              n121 = call "Stop Initiate RUN Procedure.vi"("error in (no error)"=w428, "Tamer in"=w427) -> ("error out"=w431:errorcluster, "Tamer out"=w432:refnum<class "Tamer.lvclass">)  [unwired: 8 in]
            }
          }
          n122 = Merge Errors(w424, w418) -> (w417:errorcluster)
        }
        frame "Update from Monkey" {
          n123 = Variant To Data(error in=w438, type=T14 {"Monkey ID"="", "Monkey Status"=enum."Init", "Scripts left"=0, "ETA"="", "Current Action"="", "Report from previous RUNs"="", "Skipped RUNs"=refnum} ("Monkey Status Message"), Variant=w440) -> (data=w433:T14, error out=w434:errorcluster)
          n124 = case shown="No Error" w434 {
            selector: w434 -> [w450 w500]
            tunnel: [w443 w498] -> w437
            tunnel: [w442 w499] -> w436
            tunnel: w435 -> [w451 w498]
            tunnel: w433 -> [w449 _]
            frame No Error {
              n125 = Unbundle By Name(w449) -> ("Monkey ID"=w446:string, "Monkey Status"=w441:T15)
              n126 = call-dynamic "Process Monkey Report.vi"("error in (no error)"=w450, "Monkey Status Message"=w449, "Tamer in"=w451) -> ("error out"=w454:errorcluster, "Tamer out"=w455:refnum<class "Tamer.lvclass">)  [unwired: 7 in]
              n127 = Concatenate Strings("Received update from " ("string"), w446) -> (w448:string)
              n128 = call-dynamic "Update Action History.vi"("error in (no error)"=w454, "Action"=w448, "Tamer in"=w455) -> ("error out"=w452:errorcluster, "Tamer out"=w453:refnum<class "Tamer.lvclass">)  [unwired: 7 in]
              n129 = call-dynamic "Get Status of Monkeys.vi"("error in (no error)"=w452, "Tamer in"=w453) -> ("error out"=w456:errorcluster, "Anything running?"=w458:bool, "Tamer out"=w457:refnum<class "Tamer.lvclass">)  [unwired: 7 in]
              n130 = case shown="False" w458 {
                tunnel: w457 -> [w478 w491]
                tunnel: w456 -> [w477 w493]
                tunnel: [w468 w494] -> w445
                tunnel: [w467 w492] -> w444
                tunnel: w446 -> [w476 _]
                frame False {
                  n131 = Unbundle By Name(w478) -> ("STOPPED"=w479:bool)
                  n132 = case shown="True" w479 {
                    tunnel: w478 -> [w483 w490]
                    tunnel: w477 -> [w482 w489]
                    tunnel: [w483 w490] -> w473
                    tunnel: [w482 w489] -> w470
                    tunnel: w476 -> [_ w485]
                    tunnel: [w480 w484] -> w469
                    frame False {
                      w480 = "All Monkeys Finished" ("Action")
                      n133 = call "Temporised Pop-up Window.vi"("error in (no error)"=w482, "Timeout"=5.0, "Text"=w480) -> ()  [unwired: 8 in, 1 out]
                    }
                    frame True {
                      n134 = call <vilib>:"Space Constant.vi"() -> ("String"=w488:string)
                      n135 = Concatenate Strings("STOPPED:" ("string"), w485, w488, " Finished" ("Action")) -> (w484:string)
                    }
                  }
                  n136 = call "Request to Guardian.vi"("error in (no error)"=w470, "Data"=FALSE, "Requests"=Requests."Update Run Status", "Father of all uServices in"=w473) -> ("error out"=w471:errorcluster, "Father of all uServices out"=w472:refnum<class "Tamer.lvclass">)  [unwired: 6 in]
                  n137 = call-dynamic "Update Action History.vi"("error in (no error)"=w471, "Action"=w469, "Tamer in"=w472) -> ("error out"=w467:errorcluster, "Tamer out"=w468:refnum<class "Tamer.lvclass">)  [unwired: 7 in]
                }
                frame True {
                  n138 = call "Request to Guardian.vi"("error in (no error)"=w493, "Data"=TRUE, "Requests"=Requests."Update Run Status", "Father of all uServices in"=w491) -> ("error out"=w492:errorcluster, "Father of all uServices out"=w494:refnum<class "Tamer.lvclass">)  [unwired: 6 in]
                }
              }
              n139 = case shown="\"Finished (with errors)\"" w441 {
                tunnel: w445 -> [w460 w464]
                tunnel: w444 -> [w459 w463]
                tunnel: [w460 w462] -> w443
                tunnel: [w459 w461] -> w442
                frame Default {
                }
                frame "Finished (with errors)" {
                  n140 = call "Request to Guardian.vi"("error in (no error)"=w463, "Data"=FALSE, "Requests"=Requests."Run Stopped with Errors", "Father of all uServices in"=w464) -> ("error out"=w461:errorcluster, "Father of all uServices out"=w462:refnum<class "Tamer.lvclass">)  [unwired: 6 in]
                }
              }
            }
            frame Error {
              # "#5207"
              n141 = call "Substitute Error.vi"("LabVIEW Object"=w498, "error in (no error)"=w500, "Error Code"=5207) -> ("error out"=w499:errorcluster)  [unwired: 8 in]
            }
          }
        }
        frame "Monkey Died" {
          n142 = Variant To Data(error in=w506, type="" ("Monkey ID"), Variant=w508) -> (data=w504:string, error out=w505:errorcluster)
          n143 = case shown="No Error" w505 {
            selector: w505 -> [w520 w537]
            tunnel: w504 -> [w517 _]
            tunnel: w503 -> [w526 w538]
            tunnel: [w509 w538] -> w502
            tunnel: [w510 w536] -> w501
            frame No Error {
              w514 = "The Stage" ("FP Item Name")
              n144 = call-poly "Get GUI Item Value.vi"("FP Item Name"=w514, "uService Template in"=w526) -> ("error out"=w525:errorcluster, "Value"=w524:variant)  [unwired: 7 in, 1 out]
              n145 = Unbundle By Name(w526) -> ("Monkeys"=w522:map{string, string[]})
              n146 = Variant To Data(error in=w525, type=T16[][] [] ("2D Synchronous Monkeys"), Variant=w524) -> (data=w519:T16[][])  [unwired: 1 out]
              n147 = Collection Size(1:w522) -> (0:w521:i32)
              n148 = call "Cast 2D to 1D.vi"("1D size"=w521, "2D Synchronous Monkeys"=w519) -> ("1D Synchronous Monkeys"=w518:T16[])
              n149 = call-dynamic "Monkey Died.vi"("error in (no error)"=w520, "Monkey ID"=w517, "Tamer in"=w526) -> ("error out"=w512:errorcluster, "Tamer out"=w513:refnum<class "Tamer.lvclass">)  [unwired: 7 in]
              n150 = for {
                tunnel: w518 -> [w534] mode=indexing
                tunnel: w517 -> [w533]
                tunnel: [w534] -> w516 mode=indexing if=w528
                # "Remove the Monkey from the GUI"
                n151 = Unbundle By Name(w534) -> ("Monkey ID"=w532:string)
                n152 = Empty String/Path?(string/path=w532) -> (empty?=w531:bool)
                n153 = Not Equal?(x=w532, y=w533) -> (x != y?=w529:bool)
                n154 = Not(x=w531) -> (.not. x?=w530:bool)
                n155 = And(x=w530, y=w529) -> (x .and. y?=w528:bool)
              }
              n156 = call-dynamic "Update Process Indicator.vi"("error in (no error)"=w512, "Tamer in"=w513) -> ("error out"=w511:errorcluster, "Tamer out"=w527:refnum<class "Tamer.lvclass">)  [unwired: 8 in]
              n157 = call "Cast 1D to 2D.vi"("1D Monkeys"=w516) -> ("2D Monkeys"=w515:T16[][])
              n158 = call "Update GUI.vi"("error in (no error)"=w511, "Data"=w515, "GUI Item Name"=w514, "uService Template in"=w527) -> ("error out"=w510:errorcluster, "uService Template out"=w509:refnum<class "Tamer.lvclass">)  [unwired: 6 in]
            }
            frame Error {
              # "#5773"
              n159 = call "Substitute Error.vi"("LabVIEW Object"=w538, "error in (no error)"=w537, "Error Code"=5773) -> ("error out"=w536:errorcluster)  [unwired: 8 in]
            }
          }
        }
        frame "Reschedule" {
          w548 = ""  # Process ID
          # "#5775"
          n160 = Variant To Data(error in=w550, type=w548, Variant=w549) -> (data=w539:string, error out=w547:errorcluster)
          n161 = case shown="\"ALL\"" w539 {
            selector: w539 -> [_ w568]
            tunnel: w543 -> [w566 w572]
            tunnel: w547 -> [w564 w571]
            tunnel: [w566 w570] -> w551
            tunnel: [w565 w567] -> w553
            tunnel: [w564 w569] -> w552
            frame "ALL" {
              n162 = Unbundle By Name(w566) -> ("Schedules"=w565:refnum<class "Schedule.lvclass">[])  [unwired: 1 out]
            }
            frame Default {
              n163 = call-dynamic "Get Schedules for the Process.vi"("error in (no error)"=w571, "Process ID"=w568, "Tamer in"=w572) -> ("error out"=w569:errorcluster, "Schedules"=w567:refnum<class "Schedule.lvclass">[], "Tamer out"=w570:refnum<class "Tamer.lvclass">)  [unwired: 5 in, 1 out]
            }
          }
          n164 = call "Message to uService.vi"("Father of all uServices in"=w551, "uService ID"="Scheduler" ("string"), "Message"="Reschedule", "Data"=w553, "error in (no error)"=w552) -> ("Father of all uServices out"=w542:refnum<class "Tamer.lvclass">, "error out"=w540:errorcluster)  [unwired: 9 in]
          n165 = call-dynamic "Get List of Monkeys in the Process.vi"("error in (no error)"=w540, "Process ID"=w539, "Tamer in"=w542) -> ("error out"=w563:errorcluster, "List of Monkeys"=w546:string[], "Tamer out"=w541:refnum<class "Tamer.lvclass">)  [unwired: 5 in, 1 out]
          n166 = call <vilib>:"Space Constant.vi"() -> ("String"=w558:string)
          n167 = call <vilib>:"1D String Array to Delimited String.vi"("delimiter"=", ", "string array"=w546) -> ("delimited string"=w544:string)  [unwired: 9 in]
          n168 = Concatenate Strings("Sending the schedule(s) from" ("string"), w558, w544) -> (w557:string)
          n169 = call-dynamic "Update Action History.vi"("error in (no error)"=w563, "Action"=w557, "Tamer in"=w541) -> ("error out"=w560:errorcluster, "Tamer out"=w562:refnum<class "Tamer.lvclass">)  [unwired: 7 in]
          n170 = call "Substitute Error.vi"("LabVIEW Object"=w562, "error in (no error)"=w560, "Error Code"=5775, "Optional String"=w544) -> ("error out"=w561:errorcluster)  [unwired: 7 in]
        }
        frame "Rerun" {
          w580 = ""  # Process ID
          # "#5774"
          n171 = Variant To Data(error in=w581, type=w580, Variant=w582) -> (data=w576:string, error out=w579:errorcluster)
          n172 = call-dynamic "Get Status of Monkeys.vi"("Tamer in"=w578) -> ("Anything running?"=w574:bool, "Tamer out"=w577:refnum<class "Tamer.lvclass">)  [unwired: 8 in, 1 out]
          n173 = Empty String/Path?(string/path=w576) -> (empty?=w575:bool)
          n174 = Or(x=w574, y=w575) -> (x .or. y?=w573:bool)
          n175 = case shown="False" w573 {
            tunnel: [w591 w626] -> w584
            tunnel: [w590 w625] -> w583
            tunnel: w579 -> [w589 w625]
            tunnel: w577 -> [w588 w626]
            tunnel: w576 -> [w587 _]
            frame False {
              n176 = case "Update Monkey status" shown="\"ALL\"" w587 {
                selector: w587 -> [w594 _]
                tunnel: [w603 w621] -> w591
                tunnel: [w601 w620] -> w590
                tunnel: w589 -> [w592 w617]
                tunnel: w588 -> [w593 w614]
                frame Default {
                  # "Update status of Monkeys in the proces"
                  n177 = call-dynamic "Get Schedules for the Process.vi"("error in (no error)"=w592, "Process ID"=w594, "Tamer in"=w593) -> ("error out"=w597:errorcluster, "Schedules"=w596:refnum<class "Schedule.lvclass">[], "Sync. Mask"=w595:T4[], "Tamer out"=w598:refnum<class "Tamer.lvclass">)  [unwired: 5 in]
                  n178 = call "Send Schedules to Monkeys.vi"("error in (no error)"=w597, "Schedules"=w596, "Sync. Mask"=w595, "Tamer in"=w598) -> ("error out"=w599:errorcluster, "Tamer out"=w600:refnum<class "Tamer.lvclass">)  [unwired: 6 in]
                  n179 = call-dynamic "Get List of Monkeys in the Process.vi"("error in (no error)"=w599, "Process ID"=w594, "Tamer in"=w600) -> ("error out"=w604:errorcluster, "List of Monkeys"=w605:string[], "Tamer out"=w606:refnum<class "Tamer.lvclass">)  [unwired: 5 in, 1 out]
                  n180 = for {
                    tunnel: w605 -> [w610] mode=indexing
                    tunnel: w604 -> [w611]
                    shift-right: [w609] -> w603
                    shift-left: w606 -> [w612]
                    tunnel: [w608] -> w602 mode=indexing
                    n181 = call-dynamic "Update Monkeys Status.vi"("Overwrite"=TRUE, "error in (no error)"=w611, "Status"=Monkey_Status."Init", "Monkey ID"=w610, "Tamer in"=w612) -> ("error out"=w608:errorcluster, "Tamer out"=w609:refnum<class "Tamer.lvclass">)  [unwired: 5 in]
                  }
                  n182 = Merge Errors(w602) -> (w601:errorcluster)
                }
                frame "ALL" {
                  # "Update status of all the Monkeys"
                  n183 = Unbundle By Name(w614) -> ("Sync. Mask"=w615:T4[], "Schedules"=w616:refnum<class "Schedule.lvclass">[])
                  n184 = call "Send Schedules to Monkeys.vi"("error in (no error)"=w617, "Schedules"=w616, "Sync. Mask"=w615, "Tamer in"=w614) -> ("error out"=w624:errorcluster, "Tamer out"=w618:refnum<class "Tamer.lvclass">)  [unwired: 6 in]
                  n185 = call-dynamic "Update Monkeys Status.vi"("Overwrite"=TRUE, "In ALL?"=TRUE, "error in (no error)"=w624, "Status"=Monkey_Status."Init", "Tamer in"=w618) -> ("error out"=w620:errorcluster, "Tamer out"=w621:refnum<class "Tamer.lvclass">)  [unwired: 5 in]
                }
              }
            }
            frame True {
            }
          }
          n186 = call "Substitute Error.vi"("LabVIEW Object"=w584, "error in (no error)"=w583, "Error Code"=5774) -> ("error out"=w586:errorcluster)  [unwired: 8 in]
        }
        frame "Stop Schedule" {
          w636 = T12 {"Gracefully"=FALSE, "Process"="ALL"} ("cluster")
          # "Check if the process is parallel and the gracefully flag is False, turn off the DAQ and request the STOP RUN"
          # "Just send stop schedule to Monkey with the gracefully flag"
          # "This is pretty much the new Stop Run"
          # "Stop the schedule"
          n187 = call-dynamic "Stop Periodic Replies Checks.vi"("Tamer in"=w627) -> ("Tamer out"=w628:refnum<class "Tamer.lvclass">)  [unwired: 9 in, 1 out]
          n188 = Variant To Data(type=w636, Variant=w632) -> (data=w637:T12, error out=w635:errorcluster)  [unwired: 1 in]
          n189 = property class="Tamer.lvclass"(reference=w628) -> (reference out=w638:refnum<class "Tamer.lvclass">, "Accessors:STOPPED"=w634:bool)  [unwired: 1 in, 1 out]
          n190 = case shown="Error .." w635 {
            tunnel: ["Stop button pressed. Sending STOP!" ("initial string") "Error occurred, sending STOP! " ("initial string")] -> w629
            frame No Error {
            }
            frame Error {
            }
          }
          n191 = Select(t=w636, s=w635, f=w637) -> (s? t:f=w633:T12)
          n192 = case shown="False" w634 {
            tunnel: w638 -> [w647 w698]
            tunnel: [w656 w698] -> w631
            tunnel: [w655 errorcluster {"status"=FALSE, "code"=0, "source"=""} ("error out")] -> w630
            tunnel: w633 -> [w654 _]
            tunnel: w629 -> [w645 _]
            frame False {
              # "Here it should send stop to whatever is still running. No point of sending to all"
              # "The schedules were not stopped yet"
              n193 = call-dynamic "Update Action History.vi"("Action"=w645, "Tamer in"=w647) -> ("Tamer out"=w646:refnum<class "Tamer.lvclass">)  [unwired: 8 in, 1 out]
              n194 = Unbundle By Name(w654) -> ("Process"=w649:string, "Gracefully"=w653:bool)
              n195 = Unbundle By Name(w646) -> ("Sync. Mask"=w643:T4[], "Sync. Process ID"=w652:string)
              n196 = Equal?(x=w652, y=w649) -> (x = y?=w641:bool)
              n197 = Equal?(x=w649, y="ALL") -> (x = y?=w642:bool)
              n198 = Empty Array?(array=w643) -> (empty?=w640:bool)
              n199 = Compound Arithmetic op=OR(w640, w641, w642) -> (w639:bool)
              n200 = case shown="False" w639 {
                selector: w639 -> [w663 w665]
                tunnel: w646 -> [w662 w664]
                tunnel: [w662 w668] -> w650
                tunnel: [errorcluster {"status"=FALSE, "code"=0, "source"=""} ("error out") w666] -> w660
                tunnel: [w663 w665] -> w648
                frame False {
                  # "Single process"
                }
                frame True {
                  # "Update stop flag"
                  n201 = call-dynamic "Write STOPPED.vi"("STOPPED"=TRUE, "Monkey in"=w664) -> ("error out"=w666:errorcluster, "Monkey out"=w668:refnum<class "Tamer.lvclass">)  [unwired: 8 in]
                }
              }
              n202 = case shown="False" w653 {
                tunnel: w650 -> [w673 w696]
                tunnel: [w671 w696] -> w659
                tunnel: w660 -> [w672 w695]
                tunnel: [w670 w695] -> w658
                tunnel: [_ TRUE] -> w644
                tunnel: w648 -> [w669 _]
                frame False {
                  # "Not gracefully. If stop is issued for all processes or synchronised process we need to handle the request of StopRun and the DAQ"
                  n203 = case shown="True" w669 {
                    tunnel: w673 -> [w675 w676]
                    tunnel: w672 -> [w674 w677]
                    tunnel: [w675 w679] -> w671
                    tunnel: [w674 w678] -> w670
                    frame False {
                    }
                    frame True {
                      # "#STOP_DAQ"
                      n204 = in-place {
                        in-place-border: w677 -> [w686]
                        in-place-border: [w685] -> w683
                        in-place-border: w676 -> [w684]
                        # "request the StopRun"
                        n205 = in-place-cluster #2(w676) -> ("StartRun/StopRun toggle"=w687:bool)
                        n206 = case shown="False" w687 {
                          tunnel: w686 -> [w689 w692]
                          tunnel: [w689 w691] -> w685
                          tunnel: w684 -> [_ w693]
                          frame False {
                          }
                          frame True {
                            # "#STOP_RUN"
                            n207 = call "Request to Guardian.vi"("error in (no error)"=w692, "Requests"=Requests."Stop RUN", "Father of all uServices in"=w693) -> ("error out"=w691:errorcluster)  [unwired: 7 in, 1 out]
                          }
                        }
                        n208 = in-place-cluster #2("StartRun/StopRun toggle"=FALSE) -> (w682:refnum<class "Tamer.lvclass">)
                      }
                      n209 = call "Message to uService.vi"("Father of all uServices in"=w682, "uService ID"="DAQ Manager", "Message"="Stop Run", "error in (no error)"=w683) -> ("Father of all uServices out"=w679:refnum<class "Tamer.lvclass">, "error out"=w678:errorcluster)  [unwired: 10 in]
                    }
                  }
                }
                frame True {
                  # "In gracefull stop we don't have to do anything. The script will return banana and the standard operation will proceed"
                }
              }
              n210 = call-dynamic "Message to All Monkeys in the Process.vi"("Tamer in"=w659, "Process ID"=w649, "Message"="Stop Schedule", "Data"=w644, "error in (no error)"=w658) -> ("Tamer out"=w656:refnum<class "Tamer.lvclass">, "error out"=w655:errorcluster)  [unwired: 9 in]
            }
            frame True {
              # "Stopped already"
            }
          }
        }
        frame "Skip Run" {
          n211 = call-dynamic "Read STOPPED.vi"("Monkey in"=w703) -> ("STOPPED"=w701:bool, "Monkey out"=w702:refnum<class "Tamer.lvclass">)  [unwired: 8 in, 1 out]
          n212 = case shown="False" w701 {
            tunnel: w707 -> [w722 w758]
            tunnel: w706 -> [w721 _]
            tunnel: w702 -> [w714 w759]
            tunnel: [w713 w759] -> w705
            tunnel: [w712 w758] -> w704
            frame False {
              w718 = T12 {"Gracefully"=FALSE, "Process"="ALL"} ("cluster")
              # "Nothing was stopped, we can send skip"
              n213 = Variant To Data(type=w718, Variant=w721) -> (data=w719:T12, error out=w720:errorcluster)  [unwired: 1 in]
              n214 = Select(t=w718, s=w720, f=w719) -> (s? t:f=w717:T12)
              n215 = Unbundle By Name(w717) -> ("Process"=w709:string, "Gracefully"=w711:bool)
              n216 = case shown="False" w711 {
                tunnel: w714 -> [w728 w757]
                tunnel: [w730 w757] -> w716
                tunnel: w722 -> [w731 w756]
                tunnel: [w729 w756] -> w715
                tunnel: w709 -> [w733 _]
                tunnel: [_ TRUE] -> w708
                frame False {
                  # "Not gracefully. If stop is issued for all processes or synchronised process we need to handle the request of StopRun and the DAQ"
                  n217 = Unbundle By Name(w728) -> ("Sync. Mask"=w724:T4[], "Sync. Process ID"=w734:string)
                  n218 = Empty Array?(array=w724) -> (empty?=w725:bool)
                  n219 = Equal?(x=w734, y=w733) -> (x = y?=w726:bool)
                  n220 = Equal?(x=w733, y="ALL") -> (x = y?=w727:bool)
                  n221 = Compound Arithmetic op=OR(w725, w726, w727) -> (w723:bool)
                  n222 = case shown="True" w723 {
                    tunnel: w728 -> [w736 w737]
                    tunnel: w731 -> [w735 w738]
                    tunnel: [w736 w740] -> w730
                    tunnel: [w735 w739] -> w729
                    frame False {
                    }
                    frame True {
                      # "#STOP_DAQ"
                      n223 = in-place {
                        in-place-border: w738 -> [w747]
                        in-place-border: [w746] -> w744
                        in-place-border: w737 -> [w745]
                        # "request the StopRun"
                        n224 = in-place-cluster #3(w737) -> ("StartRun/StopRun toggle"=w748:bool)
                        n225 = case shown="True" w748 {
                          tunnel: w747 -> [w750 w753]
                          tunnel: [w750 w752] -> w746
                          tunnel: w745 -> [_ w754]
                          frame False {
                          }
                          frame True {
                            # "#STOP_RUN"
                            n226 = call "Request to Guardian.vi"("error in (no error)"=w753, "Requests"=Requests."Stop RUN", "Father of all uServices in"=w754) -> ("error out"=w752:errorcluster)  [unwired: 7 in, 1 out]
                          }
                        }
                        n227 = in-place-cluster #3("StartRun/StopRun toggle"=FALSE) -> (w743:refnum<class "Tamer.lvclass">)
                      }
                      n228 = call "Message to uService.vi"("Father of all uServices in"=w743, "uService ID"="DAQ Manager", "Message"="Stop Run", "error in (no error)"=w744) -> ("Father of all uServices out"=w740:refnum<class "Tamer.lvclass">, "error out"=w739:errorcluster)  [unwired: 10 in]
                    }
                  }
                }
                frame True {
                  # "In gracefull skip we don't have to do anything. The script will return banana and the standard operation will proceed"
                }
              }
              n229 = call-dynamic "Message to All Monkeys in the Process.vi"("Tamer in"=w716, "Process ID"=w709, "Message"="Skip run", "Data"=w708, "error in (no error)"=w715) -> ("Tamer out"=w713:refnum<class "Tamer.lvclass">, "error out"=w712:errorcluster)  [unwired: 9 in]
            }
            frame True {
              # "Stopped, we don't have to do anything"
            }
          }
        }
        frame "Kill Process" {
          w761 = "ALL"
          n230 = Variant To Data(type=w761, Variant=w763) -> (data=w762:string, error out=w768:errorcluster)  [unwired: 1 in]
          n231 = Select(t=w761, s=w768, f=w762) -> (s? t:f=w760:string)
          n232 = call-dynamic "Kill Process.vi"("error in (no error)"=w766, "Process ID"=w760, "Tamer in"=w767) -> ("error out"=w765:errorcluster, "Tamer out"=w764:refnum<class "Tamer.lvclass">)  [unwired: 7 in]
        }
        frame "Update GV" {
          n233 = call "Generate Tamer Status.vi"("error in (no error)"=w772, "Monkey in"=w773) -> ("error out"=w769:errorcluster, "Tamer Panel"=w771:T18, "Monkey out"=w770:refnum<class "Tamer.lvclass">)  [unwired: 7 in]
          n234 = case shown="No Error" w769 {
            tunnel: w771 -> [w774 _]
            frame No Error {
              n235 = global write "Tamer GV.vi" "Tamer Panel"(w774) -> ()
            }
            frame Error {
            }
          }
        }
      }
    }
    frame Error {
    }
  }
  n236 = call-parent "Consumer.vi"("error in (no error)"=w8, "Data"="Data", "Case ID"="Case ID", "uService Template in"=w7) -> ("error out"=w3:errorcluster, "uService Template out"=w4:refnum<class "Tamer.lvclass">)  [unwired: 6 in]
  n237 = call-dynamic "Debug Info Display.vi"("Tamer in"=w4, "error in (no error)"=w3) -> ("Tamer out"=→"Tamer out":refnum<class "Tamer.lvclass">, "error out"=→"error out":errorcluster)  [unwired: 12 in]
